vi "Set Error.vi"(8 "error in":errorcluster, 9 "Log":string, 10 "HasError?":bool, 11 "error code":i32=-1) -> (0 "error out":errorcluster)   [LabVIEW 2023, in "LabVIEW RAG.lvlib"]
uses:
  LabVIEW RAG.lvlib
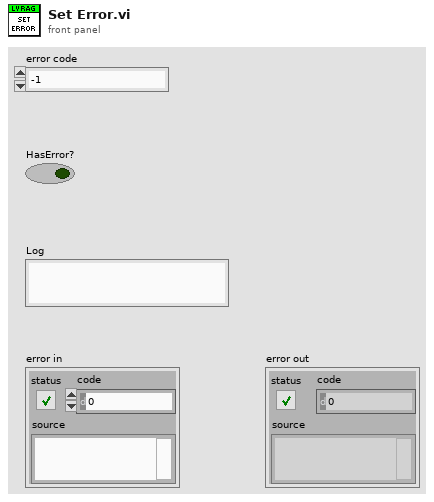
[diagram p1: front panel]
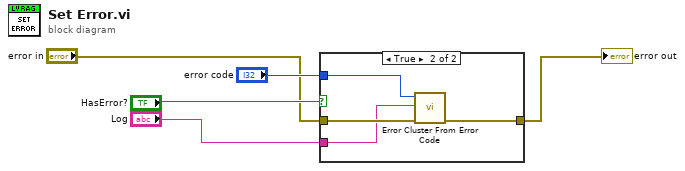
[diagram p0: block diagram]
diagram:
  n1 = case shown="True" "HasError?" {
    tunnel: "error in" -> [w6 w10]
    tunnel: [w6 w9] -> w2
    tunnel: "Log" -> [_ w8]
    tunnel: "error code" -> [_ w7]
    frame False {
    }
    frame True {
      n2 = call <vilib>:"Error Cluster From Error Code.vi"("error in (no error)"=w10, "error message (\"\")"=w8, "error code (0)"=w7) -> ("error out"=w9:errorcluster)  [unwired: 6 in]
    }
  }
  "error out" <- w2
